vi "2022_day12_sub_search_visited.vi"(9 "Val Y":i32, 10 "Val X":i32, 11 "Already Excl In.":cluster{"x":i32, "y":i32, "cost":i32}[](array[cluster])) -> (1 "Point Found?":bool, 3 "Already Excl. Out":cluster{"x":i32, "y":i32, "cost":i32}[](array[cluster]))   [LabVIEW 2021]
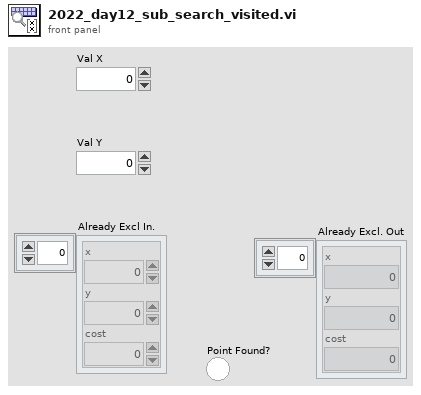
[diagram p1: front panel]
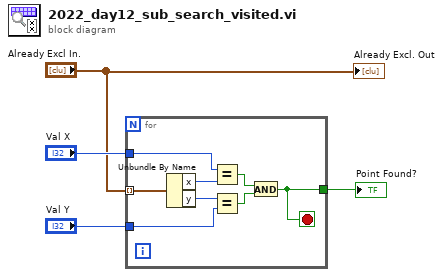
[diagram p0: block diagram]
diagram:
  n1 = for {
    tunnel: "Already Excl In." -> [w12] mode=indexing
    tunnel: "Val Y" -> [w8]
    tunnel: "Val X" -> [w10]
    tunnel: [w5] -> w1
    stop <- w5 stop-if-true
    n2 = Unbundle By Name(w12) -> ("x"=w11:i32, "y"=w9:i32)
    n3 = Equal?(x=w10, y=w11) -> (x = y?=w7:bool)
    n4 = Equal?(x=w9, y=w8) -> (x = y?=w6:bool)
    n5 = And(x=w7, y=w6) -> (x .and. y?=w5:bool)
  }
  "Point Found?" <- w1
  "Already Excl. Out" <- "Already Excl In."
